vi "Write Task Map.vi"(8 "error in (no error)":errorcluster, 10 "Task Map":T1(c390), 11 "Composite Name-Map Task in":refnum<class "Composite Name-Map Task.lvclass">) -> (0 "error out":errorcluster, 3 "Composite Name-Map Task out":refnum<class "Composite Name-Map Task.lvclass">)   [LabVIEW 2024, in "Composite Name-Map Task.lvclass"]
uses:
  Composite Name-Map Task.lvclass
  Task Ancestor/Task Ancestor.lvclass
  Composite Name-Map Task.lvclass/Composite Name-Map Task.ctl
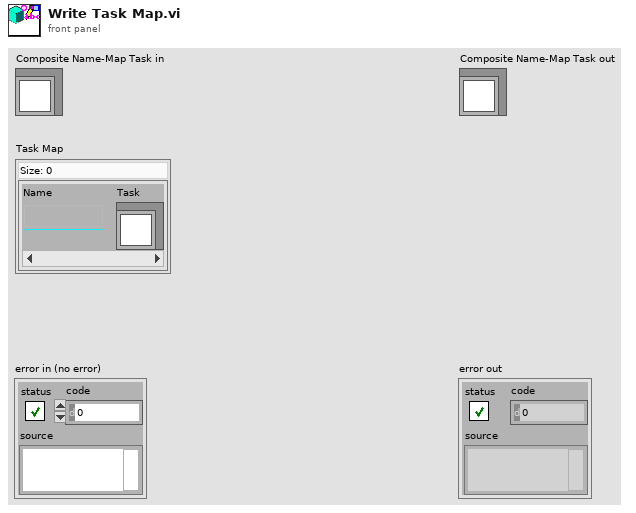
[diagram p1: front panel]
types:
  T1 = map{string, refnum<class "Task Ancestor.lvclass">}
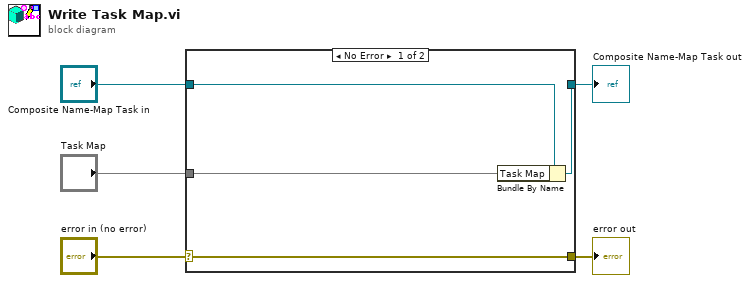
[diagram p0: block diagram]
diagram:
  n1 = case shown="No Error" "error in (no error)" {
    selector: "error in (no error)" -> [w9 w10]
    tunnel: [w9 w10] -> w4
    tunnel: [w7 w11] -> w2
    tunnel: "Composite Name-Map Task in" -> [w8 w11]
    tunnel: "Task Map" -> [w6 _]
    frame No Error {
      n2 = Bundle By Name(cluster=w8, "Task Map"=w6) -> (w7:refnum<class "Composite Name-Map Task.lvclass">)
    }
    frame Error {
    }
  }
  "error out" <- w4
  "Composite Name-Map Task out" <- w2
